vi "Channel pattern to list.vi"(11 "Pattern":u32[](array[numeric])) -> (3 "List":i32[](array[numeric]))   [LabVIEW 2020, in "Pickering.lvlib" / "PIPX40 Relay.lvclass"]
uses:
  PIPX40 Relay.lvclass
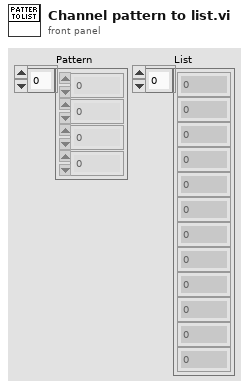
[diagram p1: front panel]
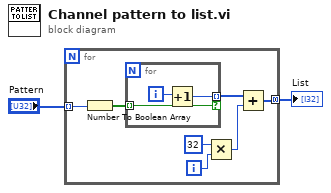
[diagram p0: block diagram]
diagram:
  n1 = for {
    tunnel: "Pattern" -> [w9] mode=indexing
    tunnel: [w3] -> w1 mode=concatenating
    i -> [w7]
    n2 = Number To Boolean Array(number=w9) -> (Boolean array=w8:bool[])
    n3 = for {
      tunnel: w8 -> [w10] mode=indexing
      tunnel: [w11] -> w5 mode=indexing if=w10
      i -> [w12]
      n4 = Increment(x=w12) -> (x+1=w11:i32)
    }
    n5 = Multiply(x=32, y=w7) -> (x*y=w4:i32)
    n6 = Add(x=w5, y=w4) -> (x+y=w3:i32[])
  }
  "List" <- w1
